vi "leds_queue.vi"() -> (0 "error out":errorcluster, 3 "queue out":refnum<queue>)   [LabVIEW 2013]
uses:
  main_machine/type_defs/led_mm.ctl
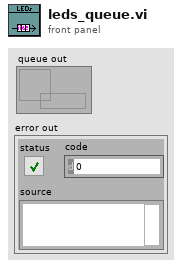
[diagram p1: front panel]
types:
  T1 = typedef "led_mm.ctl" = enum16{"INITALIZE", "START LEDS", "STROBE", "SHUTDOWN"}
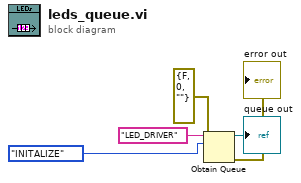
[diagram p0: block diagram]
diagram:
  n1 = Obtain Queue(name (unnamed)="LED_DRIVER", element data type=led_mm."INITALIZE", error in (no error)=errorcluster {"status"=FALSE, "code"=0, "source"=""}) -> (queue out=→"queue out":refnum<queue>, error out=→"error out":errorcluster)  [unwired: 2 in, 1 out]
